vi "Check Subject Group.vi"(11 "Subject Number":string) -> (3 "Group":string)   [LabVIEW 2020]
uses:
  <userlib>/_OpenG.lib/array/array.llb/Search 1D Array (String)__ogtk.vi
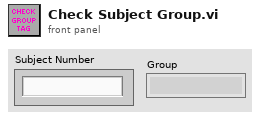
[diagram p1: front panel]
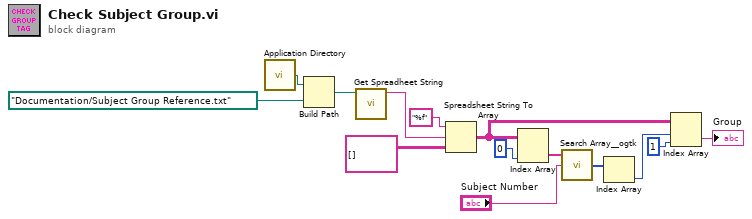
[diagram p0: block diagram]
diagram:
  n1 = call <vilib>:"Application Directory.vi"() -> ("Application Directory"=w14:path)
  n2 = Build Path(base path=w14, name or relative path=path "Documentation/Subject Group Reference.txt") -> (appended path=w12:path)
  n3 = call "Get Spreadheet String.vi"("File Path"=w12) -> ("Spreadsheet String"=w11:string)  [unwired: 9 in, 1 out]
  n4 = Spreadsheet String To Array(format string="%f", spreadsheet string=w11, array type (2D Dbl)=string[][] []) -> (array=w8:string[][])  [unwired: 1 in]
  n5 = Index Array(array=w8, index (col)=0 ("disabled index (col)")) -> (element=w6:string[])  [unwired: 1 in]
  n6 = call-poly <userlib>:"Search Array__ogtk.vi"("Array"=w6, "Element Data"="Subject Number") -> ("Indices of Elements"=w2:i32[])  [unwired: 7 in]
  n7 = Index Array(array=w2) -> (element=w1:i32)  [unwired: 1 in]
  n8 = Index Array(array=w8, index (row)=w1, index (col)=1 ("disabled index (col)")) -> (element=→"Group":string)
